vi "CD System Explorer lvlib.vi"(8 "error in (no error)":errorcluster, 9 "Action":T1) -> (0 "error out":errorcluster, 1 "Output":string)   [LabVIEW 2015]
doc: "Constants, which are necessary for the <B>CD System Explorer library</B> in the generated custom device project."
uses:
  Constants TypDef/CD System Explorer lvlib.ctl
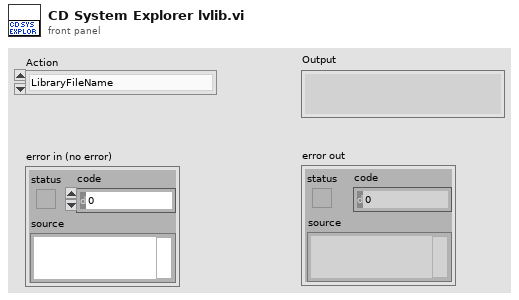
[diagram p1: front panel]
types:
  T1 = typedef "CD System Explorer lvlib.ctl" = enum16{"LibraryFileName", "LibraryFolderName", "System Explorer.FolderName", "System Explorer.Dynamically Called.FolderName", "System Explorer.Dynamically Called.Extra Pages.FolderName", "System Explorer.Dynamically Called.Extra Pages.TemplatePathAndName", "System Explorer.Dynamically Called.Main Page.VIName", "System Explorer.Dynamically Called.Main Page.TemplatePathAndName", "System Explorer.Dynamically Called.Initialization VI.VIName", "System Explorer.Dynamically Called.Initialization VI.TemplatePathAndName", "System Explorer.SubVI.FolderName", "System Explorer.Types.FolderName", "System Explorer.ActionVIOnCompile.VIName", "System Explorer.ExportConfigRTM.VIName"}
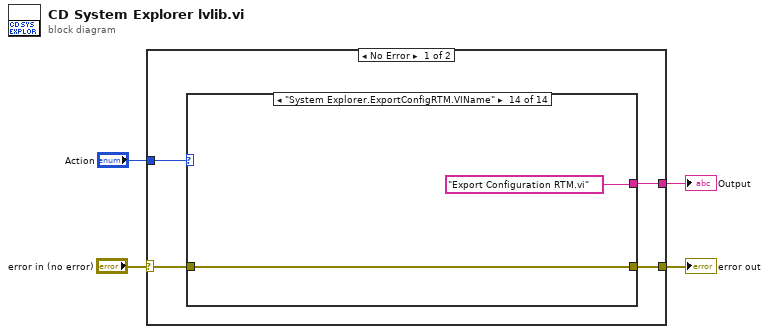
[diagram p0: block diagram]
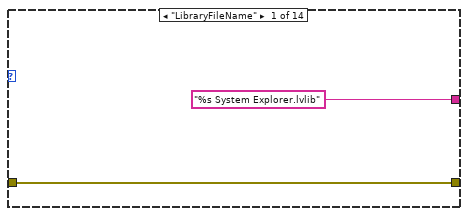
[diagram p2: hidden frame]
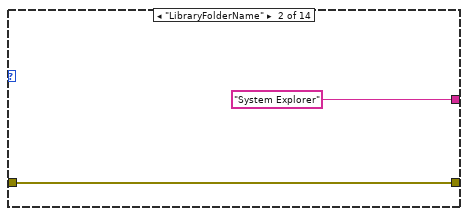
[diagram p3: hidden frame]
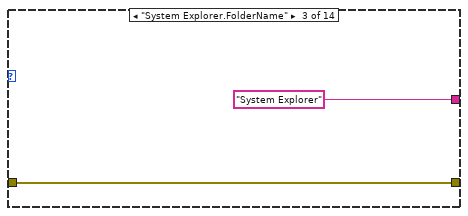
[diagram p4: hidden frame]
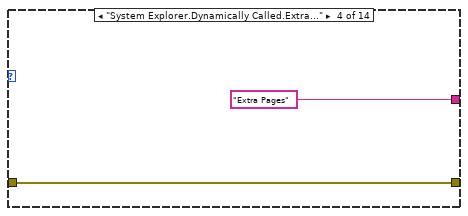
[diagram p5: hidden frame]
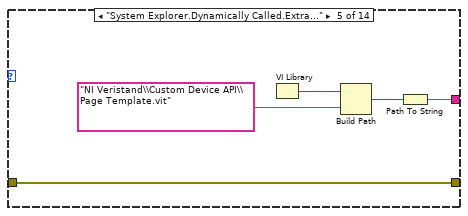
[diagram p6: hidden frame]
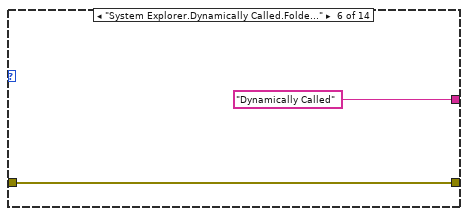
[diagram p7: hidden frame]
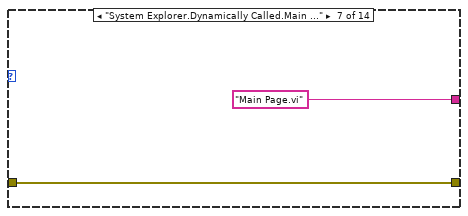
[diagram p8: hidden frame]
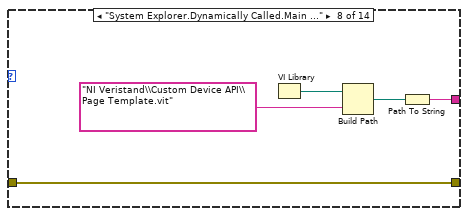
[diagram p9: hidden frame]
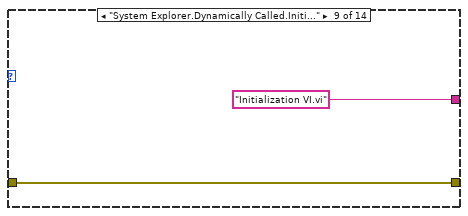
[diagram p10: hidden frame]
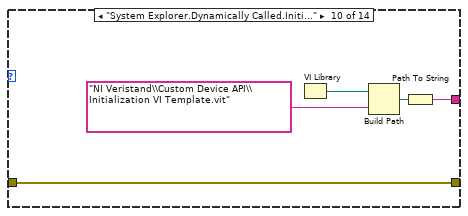
[diagram p11: hidden frame]
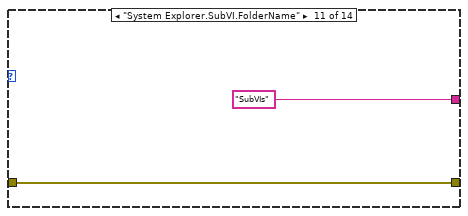
[diagram p12: hidden frame]
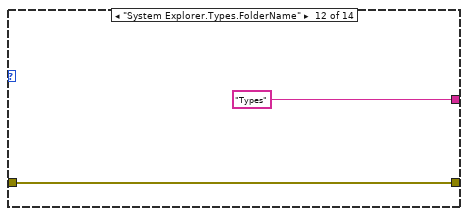
[diagram p13: hidden frame]
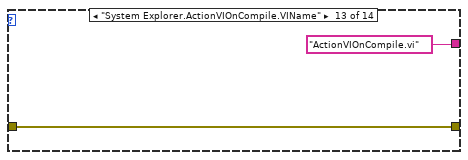
[diagram p14: hidden frame]
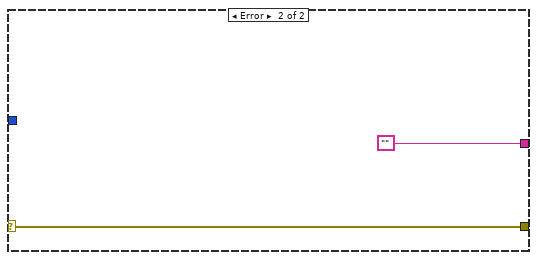
[diagram p15: hidden frame]
diagram:
  n1 = case shown="No Error" "error in (no error)" {
    selector: "error in (no error)" -> [w5 w47]
    tunnel: [w6 w47] -> w3
    tunnel: [w7 ""] -> w2
    tunnel: "Action" -> [w8 _]
    frame No Error {
      n2 = case shown="\"System Explorer.ExportConfigRTM.VIName\"" w8 {
        tunnel: ["%s System Explorer.lvlib" "System Explorer" "System Explorer" "Extra Pages" w17 "Dynamically Called" "Main Page.vi" w28 "Initialization VI.vi" w33 "SubVIs" "Types" "ActionVIOnCompile.vi" ("name or relative path") "Export Configuration RTM.vi" ("Output")] -> w7
        tunnel: [w9 w11 w13 w16 w21 w22 w24 w26 w31 w37 w38 w40 w43 w45] -> w6
        tunnel: w5 -> [w9 w11 w13 w16 w21 w22 w24 w26 w31 w37 w38 w40 w43 w45]
        frame "LibraryFileName" {
        }
        frame "LibraryFolderName" {
        }
        frame "System Explorer.FolderName" {
        }
        frame "System Explorer.Dynamically Called.Extra Pages.FolderName" {
        }
        frame "System Explorer.Dynamically Called.Extra Pages.TemplatePathAndName" {
          n3 = VI Library() -> (path=w20:path)
          n4 = Build Path(base path=w20, name or relative path="NI Veristand\\Custom Device API\\Page Template.vit") -> (appended path=w18:path)
          n5 = Path To String(path=w18) -> (string=w17:string)
        }
        frame "System Explorer.Dynamically Called.FolderName" {
        }
        frame "System Explorer.Dynamically Called.Main Page.VIName" {
        }
        frame "System Explorer.Dynamically Called.Main Page.TemplatePathAndName" {
          n6 = VI Library() -> (path=w30:path)
          n7 = Build Path(base path=w30, name or relative path="NI Veristand\\Custom Device API\\Page Template.vit") -> (appended path=w27:path)
          n8 = Path To String(path=w27) -> (string=w28:string)
        }
        frame "System Explorer.Dynamically Called.Initialization VI.VIName" {
        }
        frame "System Explorer.Dynamically Called.Initialization VI.TemplatePathAndName" {
          n9 = VI Library() -> (path=w36:path)
          n10 = Build Path(base path=w36, name or relative path="NI Veristand\\Custom Device API\\Initialization VI Template.vit") -> (appended path=w34:path)
          n11 = Path To String(path=w34) -> (string=w33:string)
        }
        frame "System Explorer.SubVI.FolderName" {
        }
        frame "System Explorer.Types.FolderName" {
        }
        frame "System Explorer.ActionVIOnCompile.VIName" {
        }
        frame "System Explorer.ExportConfigRTM.VIName" {
        }
      }
    }
    frame Error {
    }
  }
  "error out" <- w3
  "Output" <- w2
